vi "ep07_digitl_input_events.vi"() -> ()   [LabVIEW 2019]
panel:
  out "PSW3":bool
  out "PSW2":bool
  out "PSW1":bool
  out "PSW0":bool
  in  "stop":bool
  out "Service Status":bool=TRUE
  out "Port Status":bool=TRUE
  out "Information":string="ok: COM3[115200-N-8-1]\r\n"
  in  "Baud Rate":T1(ring)=enum."115200"
  in  "Port Id":T2(ring)=enum."COM3" caption="Port Name"
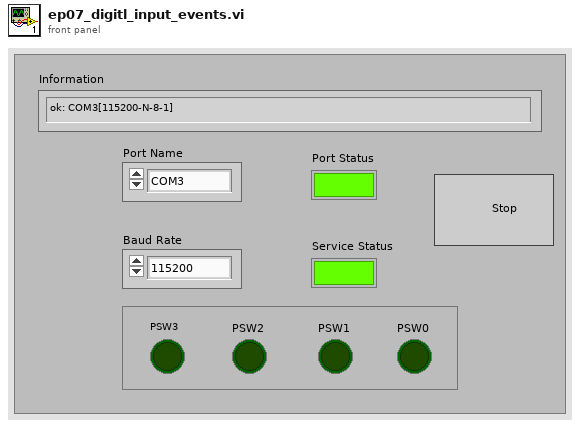
[diagram p1: front panel]
types:
  T1 = enum32{"300", "600", "1200", "2400", "4800", "9600", "14400", "19200", "28800", "38400", "56000", "57600", "115200", "128000", "256000"}
  T2 = enum8{"COM1", "COM2", "COM3", "COM4", "COM5", "COM6", "COM7", "COM8", "COM9", "COM10", "COM11", "COM12", "COM13", "COM14", "COM15", "COM16", "COM17", "COM18", "COM19", "COM20", "COM21", "COM22", "COM23", "COM24", "COM25", "COM26", "COM27", "COM28", "COM29", "COM30", "COM31", "COM32", "COM33", "COM34", "COM35", "COM36", "COM37", "COM38", "COM39", "COM40", "COM41", "COM42", "COM43", "COM44", "COM45", "COM46", "COM47", "COM48"}
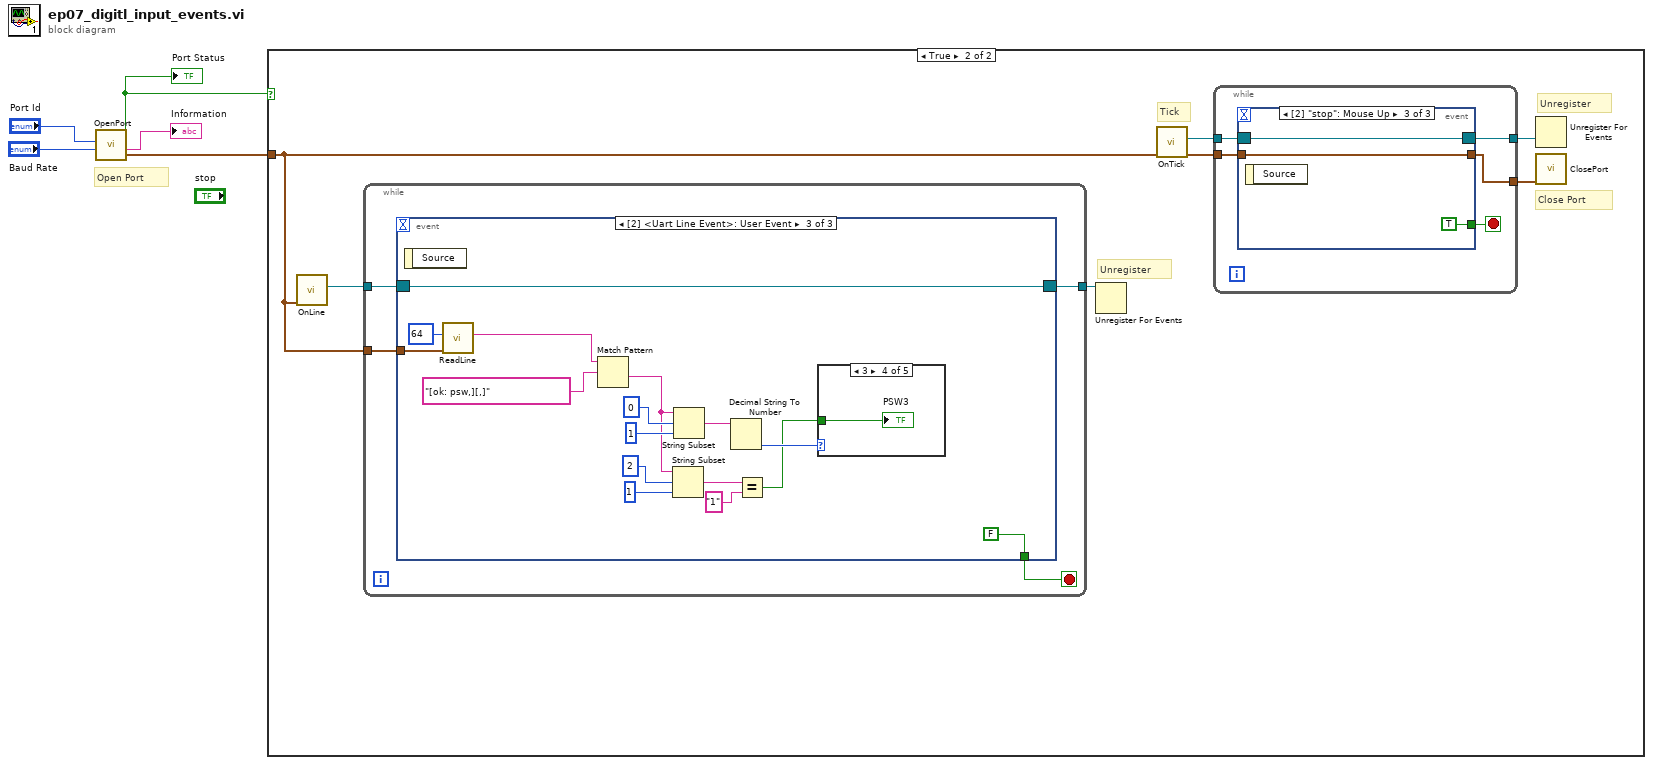
[diagram p0: block diagram]
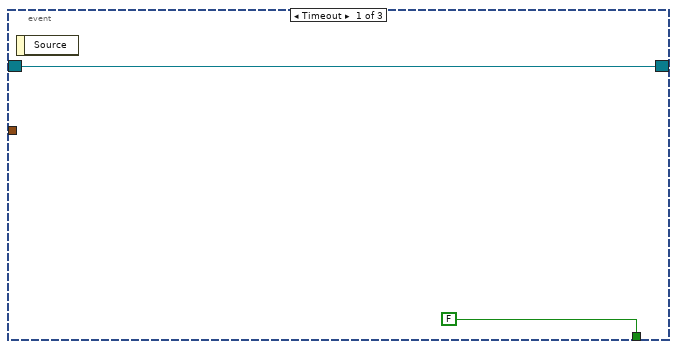
[diagram p3: hidden frame]
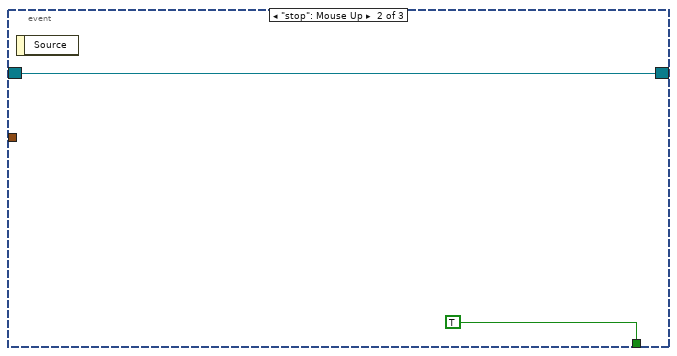
[diagram p4: hidden frame]
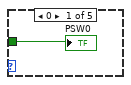
[diagram p5: hidden frame]
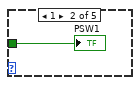
[diagram p6: hidden frame]
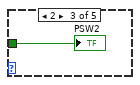
[diagram p7: hidden frame]
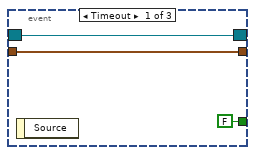
[diagram p9: hidden frame]
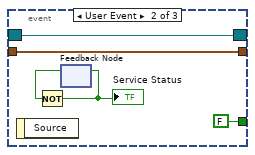
[diagram p10: hidden frame]
diagram:
  # "Open Port"
  n1 = call "OpenPort.vi"("Baud Rate Input"="Baud Rate", "Port Id Input"="Port Id") -> ("Uart Output"=w1:cluster{u64}, "Information"=→"Information":string, "Port Status"=w2:bool)  [unwired: 6 in, 1 out]
  "Port Status" <- w2
  n2 = case shown="True" w2 {
    tunnel: w1 -> [_ w6]
    frame False {
      # "Do nothing"
    }
    frame True {
      # "Unregister"
      # "Unregister"
      # "Close Port"
      # "Tick"
      n3 = call "OnLine.vi"("Uart Input"=w6) -> ("On Line Event"=w8:refnum<event-registration>)  [unwired: 8 in, 2 out]
      n4 = while {
        tunnel: w8 -> [w15]
        tunnel: [w14] -> w7
        tunnel: w6 -> [w13]
        stop <- w16 stop-if-true
        n5 = event shown="[2] <Uart Line Event>: User Event" {
          selector: w15 -> [w17 w19 w36]
          dyn-events: [w17 w19 w36] -> w14
          timeout: _ -> [_ _ _]
          tunnel: [FALSE TRUE FALSE] -> w16
          tunnel: w13 -> [_ _ w35]
          event Timeout {
            n6 = event-data() -> ()  [unwired: 1 in, 1 out]
          }
          event "stop": Mouse Up {
            n7 = event-data() -> ()  [unwired: 1 in, 1 out]
          }
          event User Event {
            n8 = event-data() -> ()  [unwired: 1 in, 1 out]
            n9 = call "ReadLine.vi"("Uart Input"=w35, "Buffer Size (32 bytes)"=u32 64) -> ("Line String"=w32:string)  [unwired: 5 in, 4 out]
            n10 = Match Pattern(string=w32, regular expression="[ok: psw,][,]") -> (after substring=w27:string)  [unwired: 1 in, 3 out]
            n11 = String Subset(string=w27, offset (0)=2, length (rest)=1 ("length (rest)")) -> (substring=w25:string)
            n12 = String Subset(string=w27, offset (0)=0, length (rest)=1 ("length (rest)")) -> (substring=w23:string)
            n13 = Decimal String To Number(string=w23) -> (number=w22:i32)  [unwired: 2 in, 1 out]
            n14 = Equal?(x=w25, y="1") -> (x = y?=w21:bool)
            n15 = case shown="3" w22 {
              tunnel: w21 -> [w37 w38 w39 w40 _]
              frame 0 {
                "PSW0" <- w37
              }
              frame 1 {
                "PSW1" <- w38
              }
              frame 2 {
                "PSW2" <- w39
              }
              frame 3 {
                "PSW3" <- w40
              }
              frame 4, Default {
              }
            }
          }
        }
      }
      n16 = Unregister For Events(event registration refnum=w7) -> ()  [unwired: 1 in, 1 out]
      n17 = call "OnTick.vi"("Uart Input"=w6) -> ("Uart Output"=w10:cluster{u64}, "On Tick Event"=w12:refnum<event-registration>)  [unwired: 8 in, 1 out]
      n18 = while {
        tunnel: w12 -> [w44]
        tunnel: [w43] -> w11
        tunnel: w10 -> [w42]
        tunnel: [w41] -> w9
        stop <- w45 stop-if-true
        n19 = event shown="[2] \"stop\": Mouse Up" {
          selector: w44 -> [w47 w50 w55]
          dyn-events: [w47 w50 w55] -> w43
          timeout: _ -> [_ _ _]
          tunnel: [FALSE FALSE TRUE] -> w45
          tunnel: [w46 w49 w54] -> w41
          tunnel: w42 -> [w46 w49 w54]
          event Timeout {
            n20 = event-data() -> ()  [unwired: 1 in, 1 out]
          }
          event User Event {
            n21 = event-data() -> ()  [unwired: 1 in, 1 out]
            n22 = feedback #1() -> (w52:bool)  [unwired: 1 in]
            n23 = Not(x=w52) -> (.not. x?=w51:bool)
            "Service Status" <- w51
            n24 = feedback-in #1(w51) -> ()
          }
          event "stop": Mouse Up {
            n25 = event-data() -> ()  [unwired: 1 in, 1 out]
          }
        }
      }
      n26 = Unregister For Events(event registration refnum=w11) -> ()  [unwired: 1 in, 1 out]
      n27 = call "ClosePort.vi"("Uart Input"=w9) -> ()  [unwired: 9 in, 2 out]
    }
  }
